vi "WSS Testor Project LAbview.vi"() -> ()   [LabVIEW 2025]
uses:
  <vilib>/Analysis/3filter.llb/Butterworth Filter (DBL).vi
  <vilib>/Analysis/NI_AALBase.lvlib
panel:
  out "After Noise filter 1":dbl[](graph)
  out "After Noise Filter 2":dbl[](graph)
  out "Input Waveform":dynamicdata(graph)
  out "Pass/Fail":bool
  out "Frequency":dbl
  out "vpp":dbl
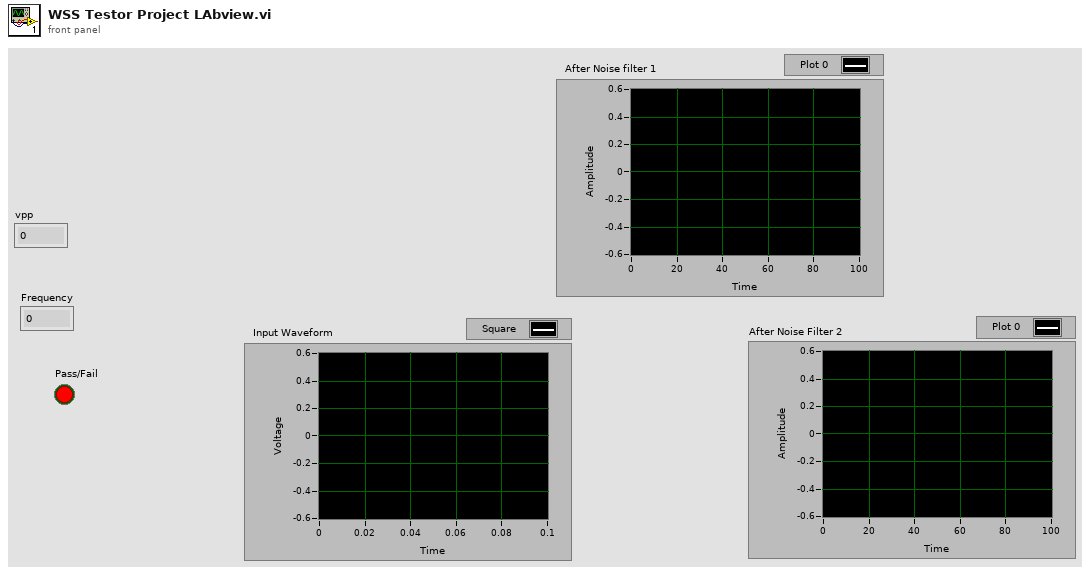
[diagram p1: front panel]
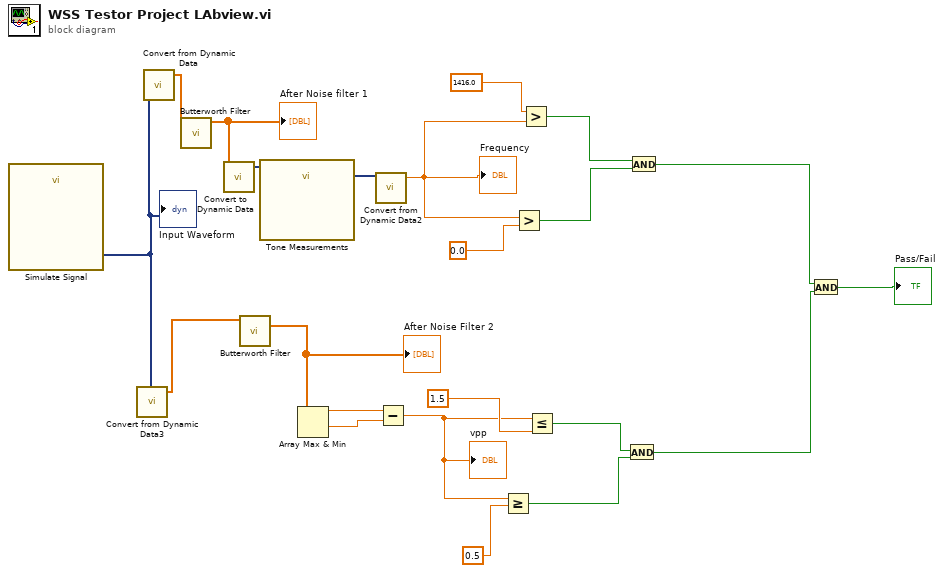
[diagram p0: block diagram]
diagram:
  n1 = call "Simulate Signal"() -> ("Square"=w8:dynamicdata)  [unwired: 14 in, 1 out]
  "Input Waveform" <- w8
  n2 = call "Convert from Dynamic Data3"("Dynamic Data Type"=w8) -> ("Array"=w4:dbl[])  [unwired: 3 in]
  n3 = call "Convert from Dynamic Data"("Dynamic Data Type"=w8) -> ("Array"=w7:dbl[])  [unwired: 3 in]
  n4 = call-poly <vilib>:"Butterworth Filter.vi"("X"=w7) -> ("Filtered X"=w5:dbl[])  [unwired: 7 in, 1 out]
  "After Noise filter 1" <- w5
  n5 = call "Convert to Dynamic Data"("Array"=w5) -> ("Dynamic Data Type"=w6:dynamicdata)  [unwired: 3 in]
  n6 = call-poly <vilib>:"Butterworth Filter.vi"("X"=w4) -> ("Filtered X"=w3:dbl[])  [unwired: 7 in, 1 out]
  "After Noise Filter 2" <- w3
  n7 = call "Tone Measurements"("Signals"=w6) -> ("Frequency"=w13:dynamicdata)  [unwired: 7 in, 3 out]
  n8 = Array Max & Min(array=w3) -> (max value=w2:dbl, min value=w1:dbl)  [unwired: 2 out]
  n9 = call "Convert from Dynamic Data2"("Dynamic Data Type"=w13) -> ("Scalar"=w12:dbl)  [unwired: 3 in]
  "Frequency" <- w12
  n10 = Subtract(x=w2, y=w1) -> (x-y=w19:dbl)
  "vpp" <- w19
  n11 = Greater Or Equal?(x=w19, y=0.5) -> (x >= y?=w21:bool)
  n12 = Greater?(x=w12, y=0.0) -> (0:w14:bool)
  n13 = Greater?(x=1416.0, y=w12) -> (0:w17:bool)
  n14 = Less Or Equal?(x=w19, y=1.5) -> (x <= y?=w22:bool)
  n15 = And(x=w22, y=w21) -> (x .and. y?=w10:bool)
  n16 = And(x=w17, y=w14) -> (x .and. y?=w11:bool)
  n17 = And(x=w11, y=w10) -> (x .and. y?=→"Pass/Fail":bool)
